vi "WPI_CANTalonSRX_CallbackSetOutput.vi"(8 "error in":errorcluster, 9 "Parameter Slot":u8, 10 "Output":dbl, 11 "MotorControlDevRef":T1={"DeviceStatus"={"status"=FALSE, "code"=0, "source"=""}, "Type"=enum."PWM", "PWM"={"PWM Channel"=enum."Invalid", "DeadBand"={"Name"="", "maxPositivePwm"=0, "minPositivePwm"=0, "centerPwm"=0, "maxNegativePwm"=0, "minNegativePwm"=0, "angularRange"=0}}, "CAN"={"Device Number"=0, "SetOutput VI Ref"=variant(enum8{"Percent VBus", "Current", "Speed", "Position", "Voltage"} enum."Percent VBus"), "GetOutput VI Ref"=variant(refnum<k1> refnum), "Enable VI Ref"=variant(dbl 12.0), "Disable VI Ref"=variant(enum8{"Percent VBus", "Speed", "Position", "Slave", "Unchanged / Invalid", "Voltage Compensation", "Current", "Motion Profile"} enum."Percent VBus"), "Data"=variant}, "Invert"=FALSE}) -> (0 "error out":errorcluster, 2 "Motor Output":dbl, 3 "MotorControlDevRef":T1={"DeviceStatus"={"status"=FALSE, "code"=0, "source"=""}, "Type"=enum."PWM", "PWM"={"PWM Channel"=enum."Invalid", "DeadBand"={"Name"="", "maxPositivePwm"=0, "minPositivePwm"=0, "centerPwm"=0, "maxNegativePwm"=0, "minNegativePwm"=0, "angularRange"=0}}, "CAN"={"Device Number"=0, "SetOutput VI Ref"=variant(enum8{"Percent VBus", "Current", "Speed", "Position", "Voltage"} enum."Percent VBus"), "GetOutput VI Ref"=variant(refnum<k1> refnum), "Enable VI Ref"=variant(dbl 12.0), "Disable VI Ref"=variant(enum8{"Percent VBus", "Speed", "Position", "Slave", "Unchanged / Invalid", "Voltage Compensation", "Current", "Motion Profile"} enum."Percent VBus"), "Data"=variant}, "Invert"=FALSE})   [LabVIEW 2016]
doc: "Specifies the output value or set-point for the motor controller.\n\nIf you use a motor controller connected to PWM, the scaled value can range from -1.0 to 1.0.\n\nIf you use a CAN Jaguar, the scale and the units depend on the mode the Jaguar is in. In <B>Percent VBus</B> mode, the range is the same as the PWM interface. In <B>Voltage</B>, <B>Current</B>, <B>Speed</B>, and <B>Position</B> modes, the <B>Output</B> is specified in engineering units (Volts, Amps, Rotations/Minute, and Rotations respectively).\n\nIf you use a CAN Talon SRX, the scale and the units depend on the mode the Talon SRXis in. In <B>Percent VBus</B> mode, the range is the same as the PWM interface. In <B>Speed</B>, and <B>Position</B> modes, the <B>Output</B> is specified in raw sensor units (ticks and ticks / 100 ms respectively).\n\nThis software is licensed. Open the labview\\readme\\WPI Robotics Library Open Source License.txt file for more information."
uses:
  <vilib>/Rock Robotics/WPI/MotorControl/WPI_MotorControlDeviceRef.ctl
  <vilib>/Rock Robotics/WPI/MotorControl/WPI_MotorControlType.ctl
  <vilib>/Rock Robotics/SystemInterfaces/DIO/FPGA_DIOPWMChannel.ctl
  <vilib>/Rock Robotics/WPI/PWM/WPI_PWMDeadband.ctl
  <vilib>/Rock Robotics/WPI/ThirdParty/CanMotor/CTRLib-LV-TalonSRX/CTRE_CANTalonSRX_UsageTypes.ctl
  <vilib>/Rock Robotics/WPI/MotorControl/WPI_MotorControlSafetyCheck.vi
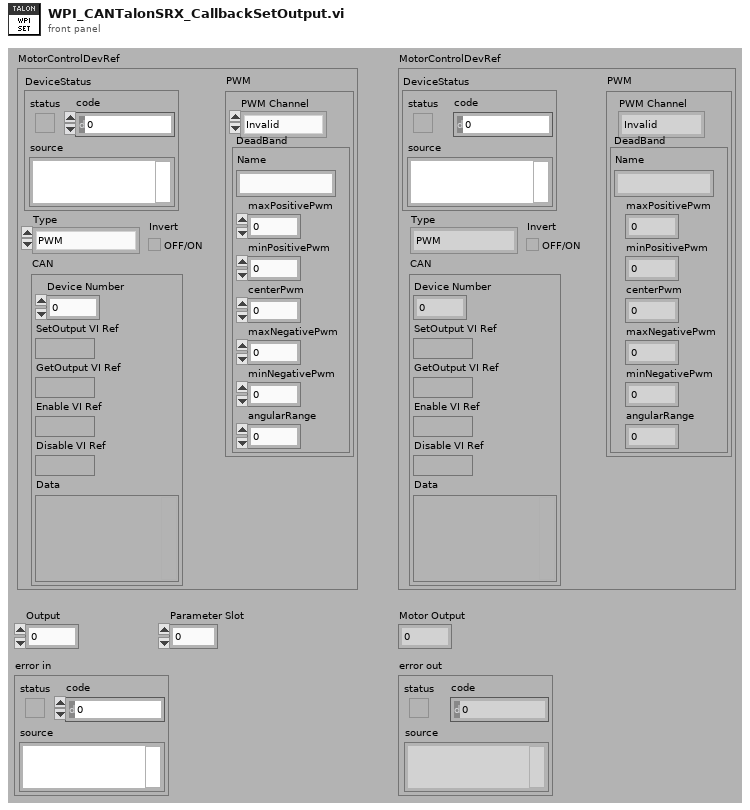
[diagram p1: front panel]
types:
  T1 = typedef "WPI_MotorControlDeviceRef.ctl" = cluster{"DeviceStatus":errorcluster, "Type":T2, "PWM":cluster{"PWM Channel":T3, "DeadBand":T4}, "CAN":cluster{"Device Number":u8, "SetOutput VI Ref":variant, "GetOutput VI Ref":variant, "Enable VI Ref":variant, "Disable VI Ref":variant, "Data":variant}, "Invert":bool}
  T2 = typedef "WPI_MotorControlType.ctl" = enum16{"PWM", "CAN"}
  T3 = typedef "FPGA_DIOPWMChannel.ctl" = enum8{"PWM 0", "PWM 1", "PWM 2", "PWM 3", "PWM 4", "PWM 5", "PWM 6", "PWM 7", "PWM 8", "PWM 9", "PWM MXP 0", "PWM MXP 1", "PWM MXP 2", "PWM MXP 3", "PWM MXP 4", "PWM MXP 5", "PWM MXP 6", "PWM MXP 7", "PWM MXP 8", "PWM MXP 9", "Invalid"}
  T4 = typedef "WPI_PWMDeadband.ctl" = cluster{"Name":string, "maxPositivePwm":i32, "minPositivePwm":i32, "centerPwm":i32, "maxNegativePwm":i32, "minNegativePwm":i32, "angularRange":u16}
  T5 = typedef "CTRE_CANTalonSRX_UsageTypes.ctl" = u32
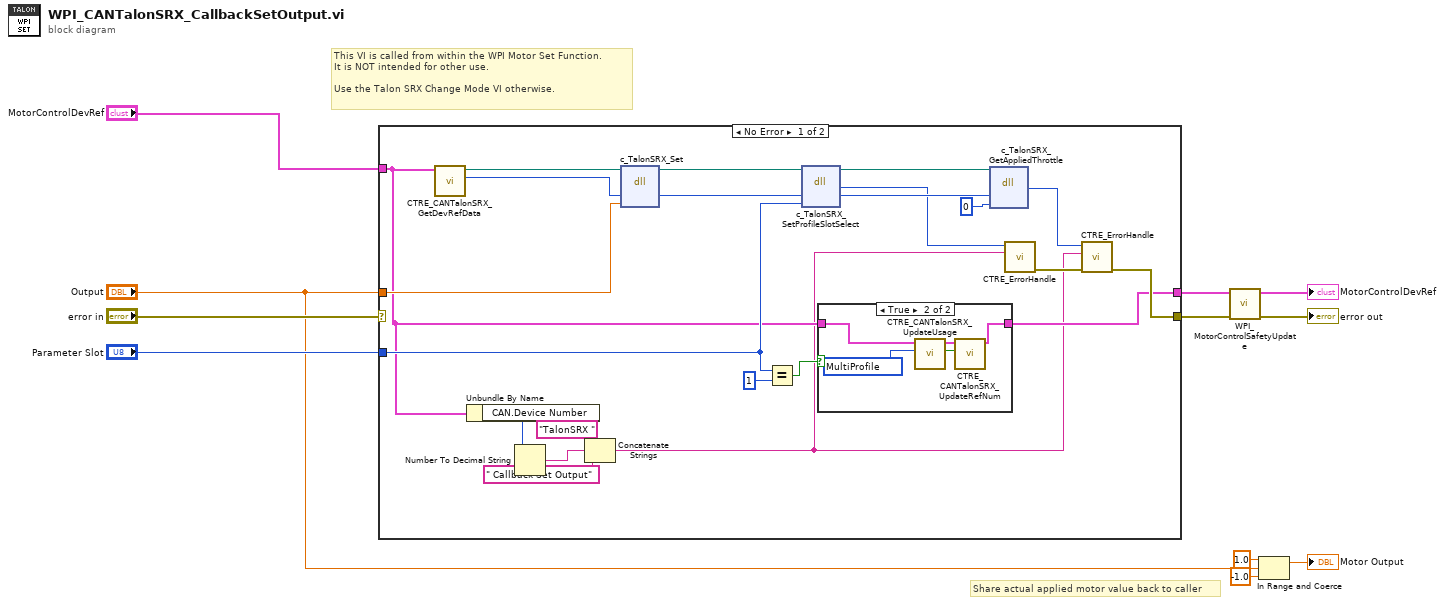
[diagram p0: block diagram]
diagram:
  # "This VI is called from within the WPI Motor Set Function.\nIt is NOT intended for other use.\n\nUse the Talon SRX Change Mode VI otherwise."
  # "Share actual applied motor value back to caller"
  n1 = case shown="No Error" "error in" {
    selector: "error in" -> [_ w41]
    tunnel: [w25 w41] -> w9
    tunnel: "MotorControlDevRef" -> [w16 w40]
    tunnel: "Output" -> [w27 _]
    tunnel: "Parameter Slot" -> [w26 _]
    tunnel: [w21 w40] -> w1
    frame No Error {
      n2 = call <vilib>:"CTRE_CANTalonSRX_GetDevRefData.vi"("MotorControlDevRef"=w16) -> ("handle"=w30:u64, "Library"=w31:path)  [unwired: 6 in, 3 out]
      n3 = Unbundle By Name(w16) -> ("CAN.Device Number"=w17:u8)
      n4 = Number To Decimal String(number=w17) -> (decimal integer string=w19:string)  [unwired: 1 in]
      n5 = Concatenate Strings("TalonSRX " ("string"), w19, " Callback Set Output" ("string")) -> (w12:string)
      n6 = dll-call lib="?" fn="c_TalonSRX_Set"(path in=w31, "handle"=w30, "value"=w27) -> (path out=w29:path, "handle"=w28:u64)  [unwired: 4 in, 1 out]
      n7 = Equal?(x=w26, y=u8 1) -> (x = y?=w32:bool)
      n8 = dll-call lib="?" fn="c_TalonSRX_SetProfileSlotSelect"(path in=w29, "handle"=w28, "profileSlot"=w26) -> (path out=w24:path, "return type"=w13:i32, "handle"=w23:u64)  [unwired: 3 in, 1 out]
      n9 = case shown="True" w32 {
        tunnel: w16 -> [w34 w39]
        tunnel: [w34 w35] -> w21
        frame False {
        }
        frame True {
          w38 = T5 2147483648 items=["Default"=0, "PercentVbus"=1, "Position"=2, "Speed"=4, "Current"=8, "Voltage"=16, "Follower"=32, "MotionProfile"=64, "MotionMagic"=128, "VRampRate"=4194304, "CurrentLimit"=8388608, "ZeroSensorI"=16777216, "ZeroSensorF"=33554432, "ZeroSensorR"=67108864, "ForwardLimitSwitch"=134217728, "ReverseLimitSwitch"=268435456, "ForwardSoftLimit"=536870912, "ReverseSoftLimit"=1073741824, "MultiProfile"=2147483648] ("Usage")
          n10 = call <vilib>:"CTRE_CANTalonSRX_UpdateUsage.vi"("Usage"=w38, "CAN Talon SRX Ref"=w39) -> ("Update"=w37:bool, "CAN Talon SRX"=w36:T1)  [unwired: 8 in]
          n11 = call <vilib>:"CTRE_CANTalonSRX_UpdateRefNum.vi"("Update"=w37, "CAN Talon SRX Ref"=w36) -> ("CAN Talon SRX Ref"=w35:T1)  [unwired: 9 in]
        }
      }
      n12 = dll-call lib="?" fn="c_TalonSRX_GetAppliedThrottle"(path in=w24, "handle"=w23, "appliedThrottle"=0) -> ("return type"=w14:i32)  [unwired: 4 in, 2 out]
      n13 = call <vilib>:"CTRE_ErrorHandle.vi"("origin"=w12, "code"=w13) -> ("error out"=w15:errorcluster)  [unwired: 9 in]
      n14 = call <vilib>:"CTRE_ErrorHandle.vi"("error in"=w15, "origin"=w12, "code"=w14) -> ("error out"=w25:errorcluster)  [unwired: 8 in]
    }
    frame Error {
    }
  }
  n15 = call <vilib>:"WPI_MotorControlSafetyUpdate.vi"("error in (no error)"=w9, "MotorControlDevRef"=w1) -> ("error out"=→"error out":errorcluster, "MotorControlDevRef"=→"MotorControlDevRef":T1)  [unwired: 8 out]
  n16 = In Range and Coerce(upper limit=1.0, x="Output", lower limit=-1.0) -> (coerced(x)=→"Motor Output":dbl)  [unwired: 1 out]
